vi "Configure Device.vi"(8 "error in (no error)":errorcluster, 10 "Max Beams":dbl, 11 "Toggle 7 1.1 in":refnum<class "Toggle 7.1.lvclass">) -> (0 "error out":errorcluster, 3 "Toggle 7 1.1 out":refnum<class "Toggle 7.1.lvclass">)   [LabVIEW 2020, in "Toggle 7.1.lvclass"]
doc: "Interface for configuring the device for testing"
uses:
  Toggle 7.1.lvclass
  Controls/EFuse modes enum.ctl
  Controls/Configure decive refs cluster.ctl
  Toggle 7.1.lvclass/Toggle 7.1.ctl
  Controls/Parameter Cluster.ctl
panel:
  in  "Enable DWA":bool
  in  "DWA":enum32{"From To", "Array"}(tab)
  in  "From To Cluster DWA":cluster{"From":dbl, "To":dbl, "Step":dbl}={"From"=29.75, "To"=29.75, "Step"=0.75} {"Step" min=0.75 max=55.0 step=0.75; "To" min=23.75 max=55.0 step=0.75; "From" min=23.75 max=55.0 step=0.75}
  in  "Array DWA":dbl[](array[numeric]) min=23.75 max=55.0 step=0.75
  in  "Efuse Multiplier":T1
  in  "Enable Charge Pump":bool
  in  "Charge Pump":enum32{"From To", "Array"}(tab)
  in  "From To Cluster Charge Pump":cluster{"From":dbl, "To":dbl, "Step":dbl}={"From"=29.75, "To"=29.75, "Step"=0.75} {"Step" min=0.75 max=55.0 step=0.75; "To" min=23.75 max=55.0 step=0.75; "From" min=23.75 max=55.0 step=0.75}
  in  "Array Charge Pump":dbl[](array[numeric]) min=23.75 max=55.0 step=0.75
  in  "OK Button":bool
  in  "Enable Register 3":bool
  in  "Register 3":enum32{"From To", "Array"}(tab)
  in  "From To Cluster Register 3":cluster{"From":dbl, "To":dbl, "Step":dbl} {"Step" min=0.375 max=7.375 step=0.375; "To" min=0.0 max=7.375 step=0.375; "From" min=0.0 max=7.375 step=0.375}
  in  "Array Register 3":dbl[](array[numeric]) min=0.0 max=7.375 step=0.375
  in  "Enable Register 2":bool
  in  "Register 2":enum32{"From To", "Array"}(tab)
  in  "From To Cluster Register 2":cluster{"From":dbl, "To":dbl, "Step":dbl} {"Step" min=0.375 max=7.375 step=0.375; "To" min=0.0 max=7.375 step=0.375; "From" min=0.0 max=7.375 step=0.375}
  in  "Array Register 2":dbl[](array[numeric]) min=0.0 max=7.375 step=0.375
  in  "Enable Register 1":bool
  in  "Register 1":enum32{"From To", "Array"}(tab)
  in  "From To Cluster Register 1":cluster{"From":dbl, "To":dbl, "Step":dbl} {"Step" min=0.125 max=7.375 step=0.125; "To" min=0.0 max=7.375 step=0.125; "From" min=0.0 max=7.375 step=0.125}
  in  "Array Register 1":dbl[](array[numeric]) min=0.0 max=7.375 step=0.125
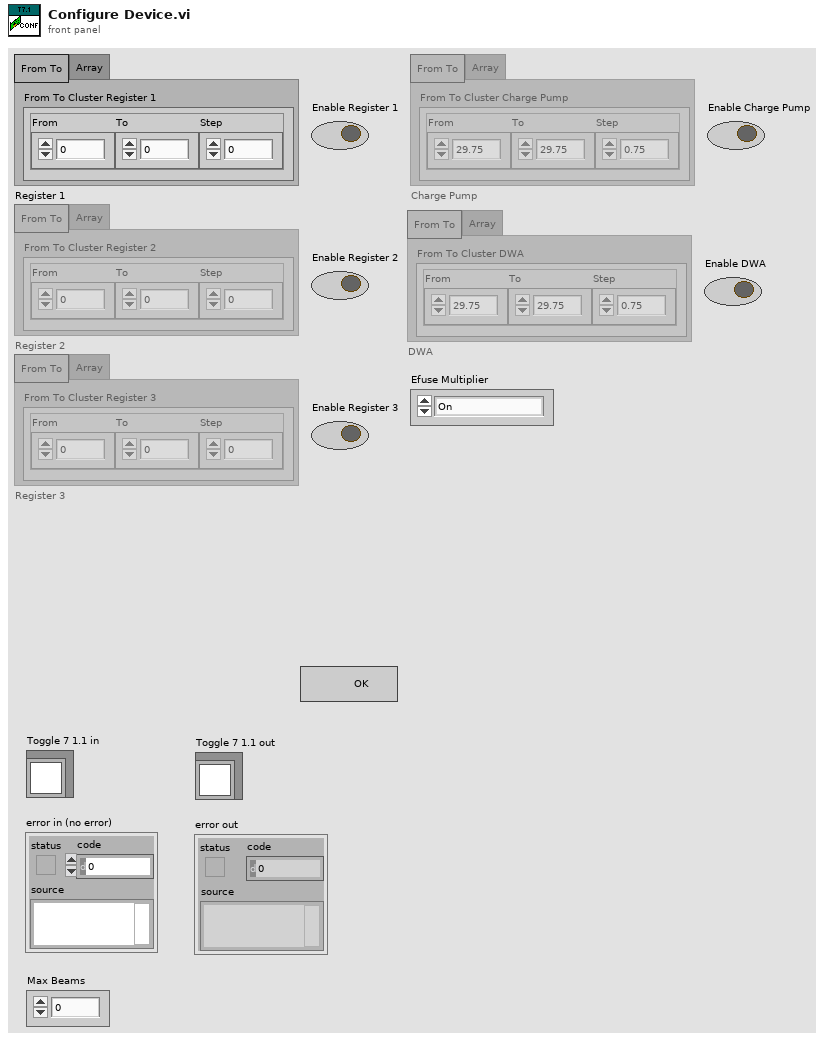
[diagram p1: front panel]
types:
  T1 = typedef "Toggle 7.1.lvclass/EFuse modes enum.ctl" = enum16{"On", "Off", "Both On and Off"}
  T2 = typedef "Toggle 7.1.lvclass/Configure decive refs cluster.ctl" = cluster{"Enable Register 1":refnum<vi>, "Register 1":refnum<vi>, "Array Register 1":refnum<vi>, "From To Cluster Register 1":refnum<vi>, "Enable Register 2":refnum<vi>, "Register 2":refnum<vi>, "Array Register 2":refnum<vi>, "From To Cluster Register 2":refnum<vi>, "Enable Register 3":refnum<vi>, "Register 3":refnum<vi>, "Array Register 3":refnum<vi>, "From To Cluster Register 3":refnum<vi>, "Enable Charge Pump":refnum<vi>, "Charge Pump":refnum<vi>, "Array Charge Pump":refnum<vi>, "From To Cluster Charge Pump":refnum<vi>, "From To Cluster DWA":refnum<vi>, "Array DWa":refnum<vi>, "Charge DWA":refnum<vi>, "Enable DWA":refnum<vi>, "Efuse Multiplier":refnum<vi>}
  T3 = typedef "Toggle 7.1.lvclass/Parameter Cluster.ctl" = cluster{"Enable":bool, "Register Number":u32, "Use Array":bool, "Array":dbl[], "To From Cluster":cluster{"From":dbl, "To":dbl, "Step":dbl}}
  T4 = enum8{"Enabled", "Disabled", "Disabled and Grayed Out"}
  T5 = typedef "Device.lvclass/Device Information Cluster.ctl" = cluster{"Device Info":string[][], "Default Values":T6[], "Fetched info":string[][]}
  T6 = typedef "PIC-Device.lvclass/Register to Write.ctl" = cluster{"Register":u32, "Value":u32, "Dev Address":u32, "Physical Adress":u32}
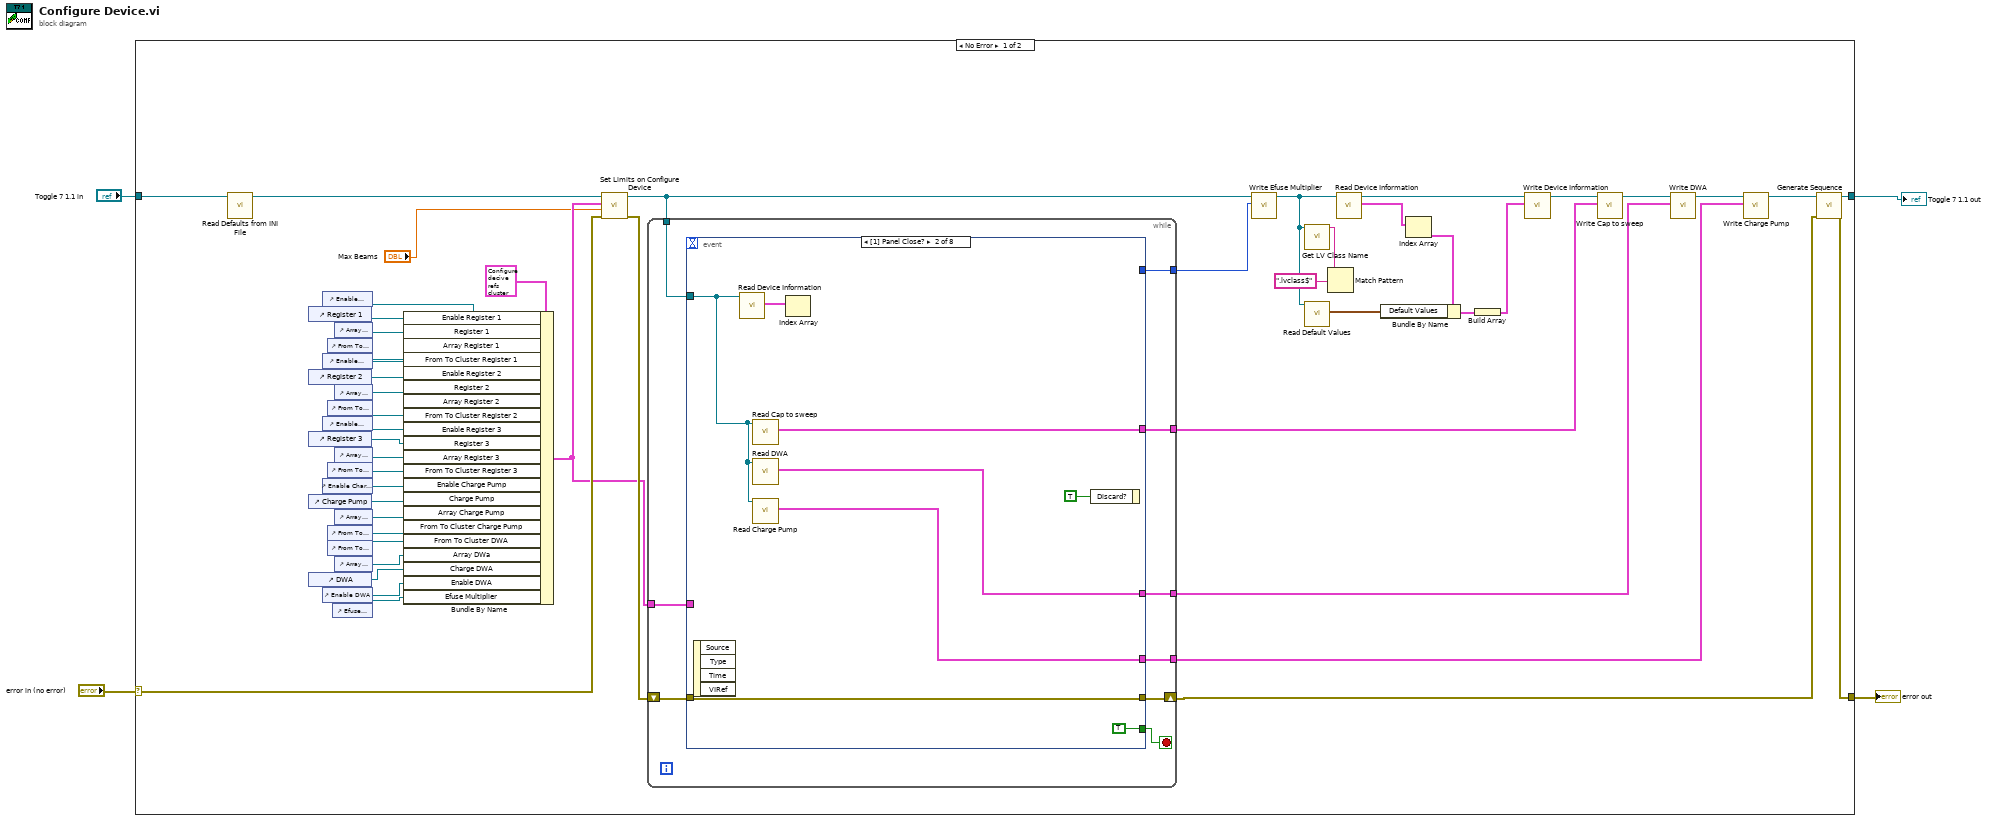
[diagram p0: block diagram]
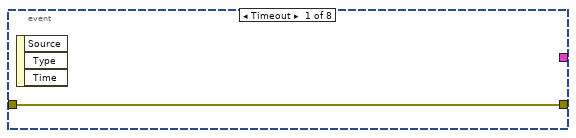
[diagram p2: hidden frame]
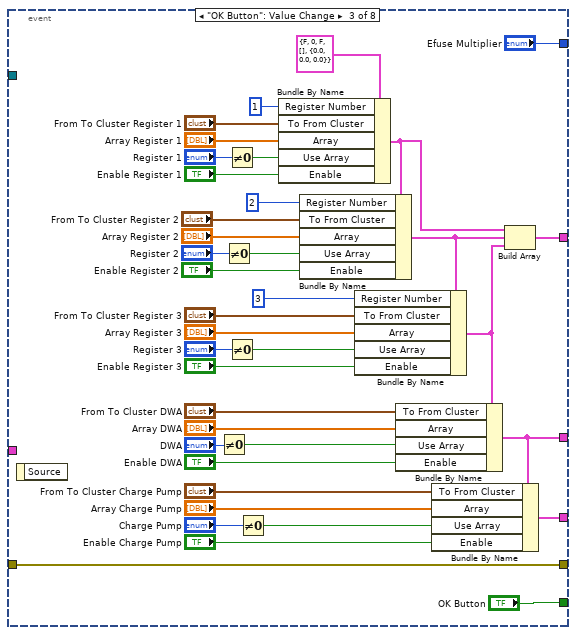
[diagram p3: hidden frame]
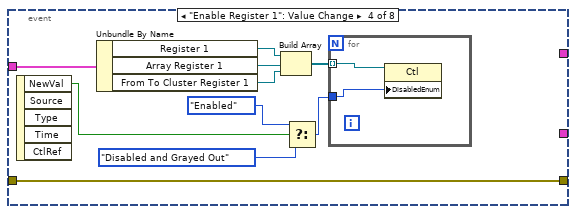
[diagram p4: hidden frame]
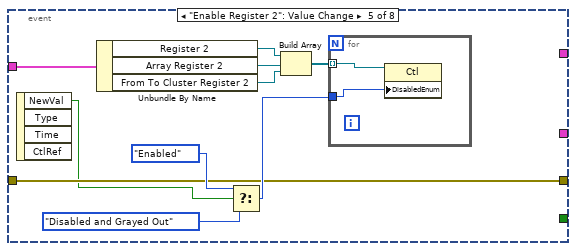
[diagram p5: hidden frame]
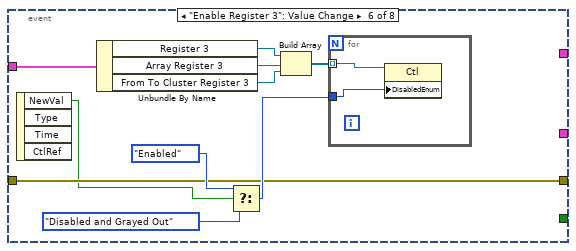
[diagram p6: hidden frame]
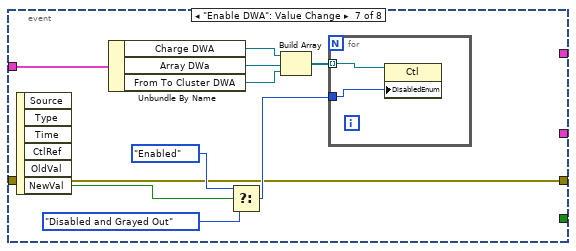
[diagram p7: hidden frame]
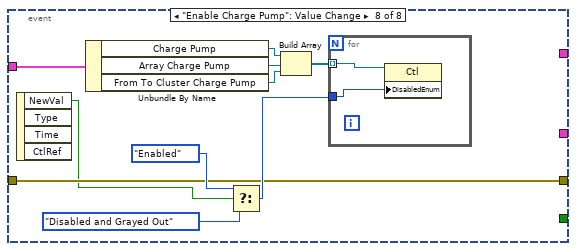
[diagram p8: hidden frame]
diagram:
  n1 = case shown="No Error" "error in (no error)" {
    selector: "error in (no error)" -> [w35 w171]
    tunnel: "Toggle 7 1.1 in" -> [w31 w170]
    tunnel: [w26 w171] -> w2
    tunnel: [w28 w170] -> w1
    frame No Error {
      n2 = call "Read Defaults from INI File.vi"("Toggle 7.1 in"=w31) -> ("Toggle 7.1 out"=w30:refnum<class "Toggle 7.1.lvclass">)  [unwired: 9 in, 1 out]
      n3 = control-ref of="Register 1"() -> (w50:refnum<vi>)
      n4 = control-ref of="Register 2"() -> (w46:refnum<vi>)
      n5 = control-ref of="Register 3"() -> (w42:refnum<vi>)
      n6 = control-ref of="Charge Pump"() -> (w38:refnum<vi>)
      n7 = control-ref of="DWA"() -> (w12:refnum<vi>)
      n8 = control-ref of="Enable Register 1"() -> (w51:refnum<vi>)
      n9 = control-ref of="Enable Register 2"() -> (w47:refnum<vi>)
      n10 = control-ref of="Enable Register 3"() -> (w43:refnum<vi>)
      n11 = control-ref of="Enable Charge Pump"() -> (w39:refnum<vi>)
      n12 = control-ref of="Enable DWA"() -> (w11:refnum<vi>)
      n13 = control-ref of="From To Cluster Register 1"() -> (w48:refnum<vi>)
      n14 = control-ref of="From To Cluster Register 2"() -> (w44:refnum<vi>)
      n15 = control-ref of="From To Cluster Register 3"() -> (w40:refnum<vi>)
      n16 = control-ref of="From To Cluster Charge Pump"() -> (w36:refnum<vi>)
      n17 = control-ref of="From To Cluster DWA"() -> (w14:refnum<vi>)
      n18 = control-ref of="Efuse Multiplier"() -> (w18:refnum<vi>)
      n19 = control-ref of="Array Register 1"() -> (w49:refnum<vi>)
      n20 = control-ref of="Array Register 2"() -> (w45:refnum<vi>)
      n21 = control-ref of="Array Register 3"() -> (w41:refnum<vi>)
      n22 = control-ref of="Array Charge Pump"() -> (w37:refnum<vi>)
      n23 = control-ref of="Array DWA"() -> (w13:refnum<vi>)
      n24 = Bundle By Name(cluster=T2 {"Enable Register 1"=refnum, "Register 1"=refnum, "Array Register 1"=refnum, "From To Cluster Register 1"=refnum, "Enable Register 2"=refnum, "Register 2"=refnum, "Array Register 2"=refnum, "From To Cluster Register 2"=refnum, "Enable Register 3"=refnum, "Register 3"=refnum, "Array Register 3"=refnum, "From To Cluster Register 3"=refnum, "Enable Charge Pump"=refnum, "Charge Pump"=refnum, "Array Charge Pump"=refnum, "From To Cluster Charge Pump"=refnum, "From To Cluster DWA"=refnum, "Array DWa"=refnum, "Charge DWA"=refnum, "Enable DWA"=refnum, "Efuse Multiplier"=refnum}, "Enable Register 1"=w51, "Register 1"=w50, "Array Register 1"=w49, "From To Cluster Register 1"=w48, "Enable Register 2"=w47, "Register 2"=w46, "Array Register 2"=w45, "From To Cluster Register 2"=w44, "Enable Register 3"=w43, "Register 3"=w42, "Array Register 3"=w41, "From To Cluster Register 3"=w40, "Enable Charge Pump"=w39, "Charge Pump"=w38, "Array Charge Pump"=w37, "From To Cluster Charge Pump"=w36, "From To Cluster DWA"=w14, "Array DWa"=w13, "Charge DWA"=w12, "Enable DWA"=w11, "Efuse Multiplier"=w18) -> (w33:T2)
      n25 = call "Set Limits on Configure Device.vi"("error in (no error)"=w35, "Max Beams"="Max Beams", "cluster"=w33, "Toggle 7.1 in"=w30) -> ("error out"=w34:errorcluster, "Toggle 7.1 out"=w9:refnum<class "Toggle 7.1.lvclass">)  [unwired: 6 in]
      n26 = while {
        shift-right: [w60] -> w27
        shift-left: w34 -> [w59]
        tunnel: w33 -> [w61]
        tunnel: [w58] -> w52
        tunnel: [w57] -> w32
        tunnel: [w56] -> w25
        tunnel: [w55] -> w15
        tunnel: w9 -> [w54]
        stop <- w62 stop-if-true
        n27 = event shown="[1] Panel Close?" {
          selector: _ -> [_ _ _ _ _ _ _ _]
          dyn-events: _ -> [_ _ _ _ _ _ _ _]
          timeout: _ -> [_ _ _ _ _ _ _ _]
          tunnel: [_ TRUE ("OK Button") "OK Button" _ _ _ _ _] -> w62
          tunnel: w61 -> [_ _ _ w119 w131 w143 w155 w167]
          tunnel: [w63 w71 w108 w111 w123 w135 w147 w159] -> w60
          tunnel: w59 -> [w63 w71 w108 w111 w123 w135 w147 w159]
          tunnel: [_ w64 w89 _ _ _ _ _] -> w58
          tunnel: [_ w66 w81 _ _ _ _ _] -> w57
          tunnel: [_ _ "Efuse Multiplier" _ _ _ _ _] -> w56
          tunnel: [_ w65 w76 _ _ _ _ _] -> w55
          tunnel: w54 -> [_ w67 _ _ _ _ _ _]
          event Timeout {
            n28 = event-data() -> ()  [unwired: 1 in, 3 out]
          }
          event Panel Close? {
            n29 = event-data() -> ()  [unwired: 1 in, 4 out]
            n30 = call-dynamic "Read Device Information.vi"("Device in"=w67) -> ("Device Info"=w68:T5[])  [unwired: 8 in, 2 out]
            n31 = call-dynamic "Read Cap to sweep.vi"("Toggle 6 in"=w67) -> ("Cap to sweep"=w66:T3[])  [unwired: 9 in, 1 out]
            n32 = call "Read DWA.vi"("Toggle 7.1 in"=w67) -> ("Parameter Cluster"=w65:T3)  [unwired: 9 in, 1 out]
            n33 = call-dynamic "Read Charge Pump.vi"("Toggle 7.1 in"=w67) -> ("Parameter Cluster"=w64:T3)  [unwired: 8 in, 2 out]
            n34 = Index Array(array=w68) -> ()  [unwired: 1 in, 1 out]
            n35 = event-data("Discard?"=TRUE) -> ()  [unwired: 1 in, 1 out]
          }
          event "OK Button": Value Change {
            n36 = event-data() -> ()  [unwired: 1 in, 1 out]
            n37 = Not Equal To 0?(x="DWA") -> (x != 0?=w103:bool)
            n38 = Not Equal To 0?(x="Register 2") -> (x != 0?=w98:bool)
            n39 = Not Equal To 0?(x="Register 1") -> (x != 0?=w93:bool)
            n40 = Not Equal To 0?(x="Register 3") -> (x != 0?=w102:bool)
            n41 = Not Equal To 0?(x="Charge Pump") -> (x != 0?=w107:bool)
            n42 = Bundle By Name(cluster=T3 {"Enable"=FALSE, "Register Number"=0, "Use Array"=FALSE, "Array"=[], "To From Cluster"={"From"=0.0, "To"=0.0, "Step"=0.0}} ("output cluster"), "Register Number"=u32 1, "To From Cluster"="From To Cluster Register 1", "Array"="Array Register 1", "Use Array"=w93, "Enable"="Enable Register 1") -> (w84:T3)
            n43 = Bundle By Name(cluster=w84, "Register Number"=u32 2, "To From Cluster"="From To Cluster Register 2", "Array"="Array Register 2", "Use Array"=w98, "Enable"="Enable Register 2") -> (w83:T3)
            n44 = Bundle By Name(cluster=w83, "Register Number"=u32 3, "To From Cluster"="From To Cluster Register 3", "Array"="Array Register 3", "Use Array"=w102, "Enable"="Enable Register 3") -> (w82:T3)
            n45 = Bundle By Name(cluster=w82, "To From Cluster"="From To Cluster DWA", "Array"="Array DWA", "Use Array"=w103, "Enable"="Enable DWA") -> (w76:T3)
            n46 = Bundle By Name(cluster=w76, "To From Cluster"="From To Cluster Charge Pump", "Array"="Array Charge Pump", "Use Array"=w107, "Enable"="Enable Charge Pump") -> (w89:T3)
            n47 = Build Array(w84, w83, w82) -> (w81:T3[])
          }
          event "Enable Register 1": Value Change {
            n48 = event-data() -> ("NewVal"=w110:bool)  [unwired: 1 in, 4 out]
            n49 = Unbundle By Name(w119) -> ("Register 1"=w118:refnum<vi>, "Array Register 1"=w117:refnum<vi>, "From To Cluster Register 1"=w116:refnum<vi>)
            n50 = Build Array(w118, w117, w116) -> (w115:refnum<vi>[])
            n51 = Select(t=T4."Enabled" ("Disabled"), s=w110, f=T4."Disabled and Grayed Out") -> (s? t:f=w114:T4)
            n52 = for {
              tunnel: w115 -> [w121] mode=indexing
              tunnel: w114 -> [w120]
              n53 = property class="Ctl"(reference=w121, "DisabledEnum"=w120) -> ()  [unwired: 1 in, 2 out]
            }
          }
          event "Enable Register 2": Value Change {
            n54 = event-data() -> ("NewVal"=w122:bool)  [unwired: 1 in, 3 out]
            n55 = Unbundle By Name(w131) -> ("Register 2"=w130:refnum<vi>, "Array Register 2"=w129:refnum<vi>, "From To Cluster Register 2"=w128:refnum<vi>)
            n56 = Select(t=T4."Enabled" ("Disabled"), s=w122, f=T4."Disabled and Grayed Out") -> (s? t:f=w126:T4)
            n57 = Build Array(w130, w129, w128) -> (w127:refnum<vi>[])
            n58 = for {
              tunnel: w127 -> [w133] mode=indexing
              tunnel: w126 -> [w132]
              n59 = property class="Ctl"(reference=w133, "DisabledEnum"=w132) -> ()  [unwired: 1 in, 2 out]
            }
          }
          event "Enable Register 3": Value Change {
            n60 = event-data() -> ("NewVal"=w134:bool)  [unwired: 1 in, 3 out]
            n61 = Unbundle By Name(w143) -> ("Register 3"=w142:refnum<vi>, "Array Register 3"=w141:refnum<vi>, "From To Cluster Register 3"=w140:refnum<vi>)
            n62 = Select(t=T4."Enabled" ("Disabled"), s=w134, f=T4."Disabled and Grayed Out") -> (s? t:f=w138:T4)
            n63 = Build Array(w142, w141, w140) -> (w139:refnum<vi>[])
            n64 = for {
              tunnel: w139 -> [w145] mode=indexing
              tunnel: w138 -> [w144]
              n65 = property class="Ctl"(reference=w145, "DisabledEnum"=w144) -> ()  [unwired: 1 in, 2 out]
            }
          }
          event "Enable DWA": Value Change {
            n66 = event-data() -> ("NewVal"=w146:bool)  [unwired: 1 in, 5 out]
            n67 = Unbundle By Name(w155) -> ("Charge DWA"=w154:refnum<vi>, "Array DWa"=w153:refnum<vi>, "From To Cluster DWA"=w152:refnum<vi>)
            n68 = Select(t=T4."Enabled" ("Disabled"), s=w146, f=T4."Disabled and Grayed Out") -> (s? t:f=w150:T4)
            n69 = Build Array(w154, w153, w152) -> (w151:refnum<vi>[])
            n70 = for {
              tunnel: w151 -> [w157] mode=indexing
              tunnel: w150 -> [w156]
              n71 = property class="Ctl"(reference=w157, "DisabledEnum"=w156) -> ()  [unwired: 1 in, 2 out]
            }
          }
          event "Enable Charge Pump": Value Change {
            n72 = event-data() -> ("NewVal"=w158:bool)  [unwired: 1 in, 3 out]
            n73 = Unbundle By Name(w167) -> ("Charge Pump"=w166:refnum<vi>, "Array Charge Pump"=w165:refnum<vi>, "From To Cluster Charge Pump"=w164:refnum<vi>)
            n74 = Select(t=T4."Enabled" ("Disabled"), s=w158, f=T4."Disabled and Grayed Out") -> (s? t:f=w162:T4)
            n75 = Build Array(w166, w165, w164) -> (w163:refnum<vi>[])
            n76 = for {
              tunnel: w163 -> [w169] mode=indexing
              tunnel: w162 -> [w168]
              n77 = property class="Ctl"(reference=w169, "DisabledEnum"=w168) -> ()  [unwired: 1 in, 2 out]
            }
          }
        }
      }
      n78 = call-dynamic "Write Efuse Multiplier.vi"("Efuse Multiplier"=w25, "Toggle 6 in"=w9) -> ("Toggle 6 out"=w7:refnum<class "Toggle 7.1.lvclass">)  [unwired: 9 in]
      n79 = call <vilib>:"Get LV Class Name.vi"("object"=w7) -> ("class name"=w23:string)  [unwired: 9 in, 1 out]
      n80 = call-dynamic "Read Default Values.vi"("Toggle 7.1 in"=w7) -> ("Default Values"=w22:T6[])  [unwired: 9 in, 1 out]
      n81 = Match Pattern(string=w23, regular expression=".lvclass$") -> ()  [unwired: 1 in, 4 out]
      n82 = call-dynamic "Read Device Information.vi"("Device in"=w7) -> ("Device Info"=w8:T5[], "Device out"=w6:refnum<class "Toggle 7.1.lvclass">)  [unwired: 8 in, 1 out]
      n83 = Index Array(array=w8) -> (element=w5:T5)  [unwired: 1 in]
      n84 = Bundle By Name(cluster=w5, "Default Values"=w22) -> (w21:T5)
      n85 = Build Array(w21) -> (w20:T5[])
      n86 = call-dynamic "Write Device Information.vi"("Device Info"=w20, "Device in"=w6) -> ("Device out"=w24:refnum<class "Toggle 7.1.lvclass">)  [unwired: 8 in, 1 out]
      n87 = call-dynamic "Write Cap to sweep.vi"("Cap to sweep"=w32, "Toggle 6 in"=w24) -> ("Toggle 6 out"=w17:refnum<class "Toggle 7.1.lvclass">)  [unwired: 9 in]
      n88 = call "Write DWA.vi"("Parameter Cluster"=w15, "Toggle 7.1 in"=w17) -> ("Toggle 7.1 out"=w16:refnum<class "Toggle 7.1.lvclass">)  [unwired: 9 in]
      n89 = call-dynamic "Write Charge Pump.vi"("Parameter Cluster"=w52, "Toggle 6 in"=w16) -> ("Toggle 6 out"=w29:refnum<class "Toggle 7.1.lvclass">)  [unwired: 8 in, 1 out]
      n90 = call "Generate Sequence.vi"("error in (no error)"=w27, "Toggle 7.1 in"=w29) -> ("error out"=w26:errorcluster, "Toggle 7.1 out"=w28:refnum<class "Toggle 7.1.lvclass">)  [unwired: 8 in]
    }
    frame Error {
    }
  }
  "error out" <- w2
  "Toggle 7 1.1 out" <- w1
